vi "Quadratic Roots.vi"() -> ()   [LabVIEW 2024]
panel:
  out "Root 2":dbl
  out "Root 1":dbl
  in  "C":dbl
  in  "B":dbl
  in  "A":dbl
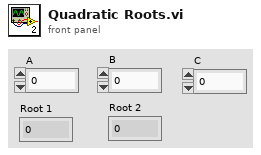
[diagram p1: front panel]
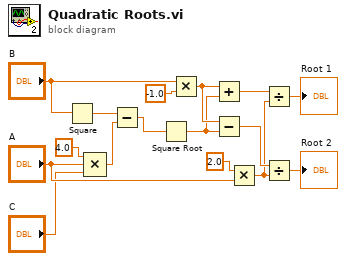
[diagram p0: block diagram]
diagram:
  n1 = Square(x="B") -> (x^2=w10:dbl)
  n2 = Compound Arithmetic op=MULTIPLY(4.0, "A", "C") -> (w9:dbl)
  n3 = Subtract(x=w10, y=w9) -> (x-y=w8:dbl)
  n4 = Square Root(x=w8) -> (sqrt(x)=w6:dbl)
  n5 = Multiply(x="B", y=-1.0) -> (x*y=w7:dbl)
  n6 = Add(x=w7, y=w6) -> (x+y=w5:dbl)
  n7 = Subtract(x=w7, y=w6) -> (x-y=w4:dbl)
  n8 = Multiply(x=2.0, y="A") -> (x*y=w3:dbl)
  n9 = Divide(x=w5, y=w3) -> (x/y=→"Root 1":dbl)
  n10 = Divide(x=w4, y=w3) -> (x/y=→"Root 2":dbl)
